vi "Filter-Init.vi"(5 "Filter":T1 {"IIR Filter Cluster"."Forward Coefficients" format="%.4f"; "IIR Filter Cluster"."Reverse Coefficients" format="%.4f"}, 9 "Sampling rate (Hz)":dbl, 11 "error in (no error)":errorcluster) -> (6 "Filter out":T1 {"IIR Filter Cluster"."Forward Coefficients" format="%.4f"; "IIR Filter Cluster"."Reverse Coefficients" format="%.4f"}, 15 "error out":errorcluster)   [LabVIEW 2020]
uses:
  Controls/Filter XCtl/Filter Data.ctl
  <vilib>/Analysis/3filter.llb/Filter Passband Type.ctl
  <vilib>/Analysis/NI_AALBase.lvlib
  Controls/Filter XCtl/Filter XCtl.xctl
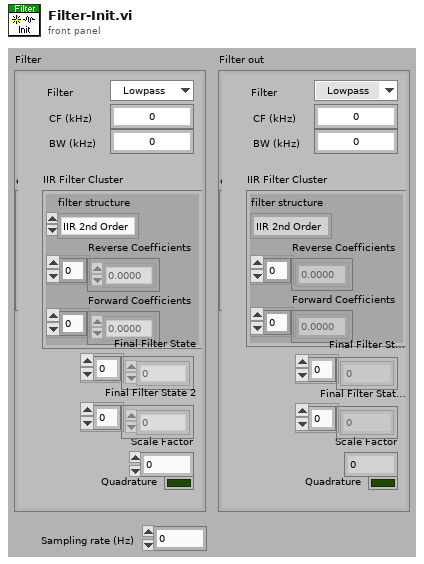
[diagram p1: front panel]
types:
  T1 = typedef "Filter XCtl.xctl/Filter Data.ctl" = cluster{"CF (kHz)":dbl, "BW (kHz)":dbl, "IIR Filter Cluster":cluster{"filter structure":enum32{"IIR 2nd Order", "IIR 4th Order"}, "Reverse Coefficients":dbl[], "Forward Coefficients":dbl[]}, "Final Filter State":dbl[], "Scale Factor":dbl, "Final Filter State 2":dbl[], "Quadrature":bool, "Type":enum16{"Lowpass", "Highpass", "Bandpass", "Bandstop", "OFF"}}
  T2 = enum16{"Lowpass", "Highpass", "Bandpass", "Bandstop", "OFF"}
  T3 = typedef "NI_AALBase.lvlib/Filter Passband Type.ctl" = enum32{"Lowpass", "Highpass", "Bandpass", "Bandstop"}
  T4 = cluster{"filter structure":enum32{"IIR 2nd Order", "IIR 4th Order"}, "Reverse Coefficients":dbl[], "Forward Coefficients":dbl[]}
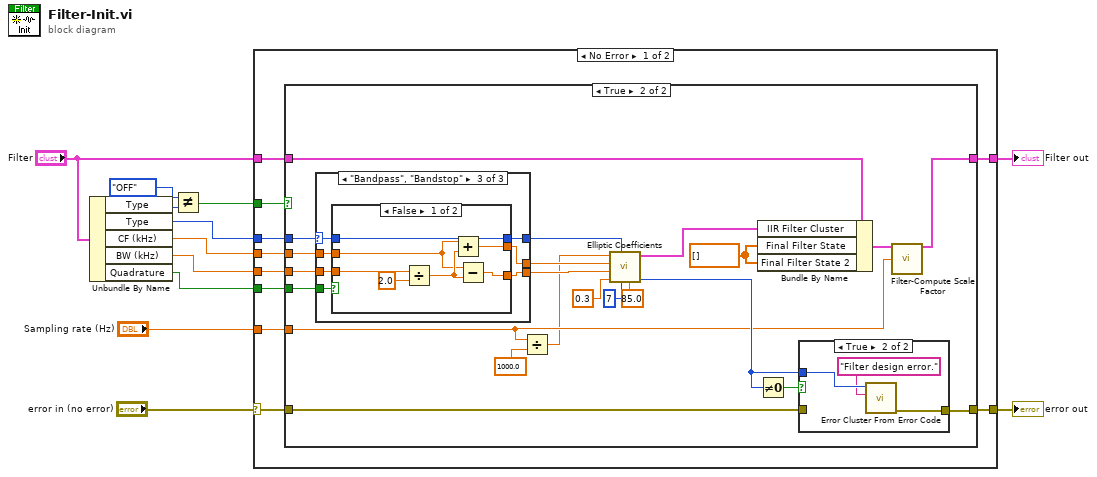
[diagram p0: block diagram]
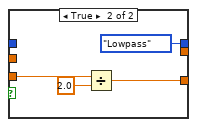
[diagram p6: hidden frame]
diagram:
  n1 = Unbundle By Name("Filter") -> ("Type"=w3:T2, "Type"=w11:T2, "CF (kHz)"=w8:dbl, "BW (kHz)"=w7:dbl, "Quadrature"=w4:bool)
  n2 = Not Equal?(x=T2."OFF", y=w3) -> (x != y?=w1:bool)
  n3 = case shown="No Error" "error in (no error)" {
    selector: "error in (no error)" -> [w15 w73]
    tunnel: w1 -> [w22 _]
    tunnel: w11 -> [w21 _]
    tunnel: "Sampling rate (Hz)" -> [w20 _]
    tunnel: "Filter" -> [w19 w74]
    tunnel: [w18 w74] -> w9
    tunnel: w8 -> [w17 _]
    tunnel: w7 -> [w16 _]
    tunnel: [w14 w73] -> w6
    tunnel: w4 -> [w13 _]
    frame No Error {
      n4 = case shown="True" w22 {
        tunnel: w21 -> [_ w31]
        tunnel: w20 -> [_ w33]
        tunnel: w19 -> [w24 w46]
        tunnel: [w24 w35] -> w18
        tunnel: w17 -> [_ w45]
        tunnel: w16 -> [_ w42]
        tunnel: w15 -> [w23 w40]
        tunnel: [w23 w39] -> w14
        tunnel: w13 -> [_ w28]
        frame False {
        }
        frame True {
          w30 = dbl[] [] ("Final Filter State")
          n5 = case shown="\"Bandpass\", \"Bandstop\"" w31 {
            selector: w31 -> [w51 w53 w56]
            tunnel: w45 -> [w52 w54 w58]
            tunnel: [w52 _ w59] -> w44
            tunnel: [_ w54 w60] -> w43
            tunnel: w42 -> [_ _ w61]
            tunnel: [w51 w53 w55] -> w29
            tunnel: w28 -> [_ _ w57]
            frame "Lowpass", Default {
            }
            frame "Highpass" {
            }
            frame "Bandpass", "Bandstop" {
              n6 = case shown="False" w57 {
                tunnel: w61 -> [w68 w71]
                tunnel: [w66 _] -> w60
                tunnel: [w65 w69] -> w59
                tunnel: w58 -> [w63 _]
                tunnel: w56 -> [w62 _]
                tunnel: [w62 Filter_Passband_Type."Lowpass" ("filter type")] -> w55
                frame False {
                  n7 = Divide(x=w68, y=2.0) -> (x/y=w64:dbl)
                  n8 = Add(x=w63, y=w64) -> (x+y=w66:dbl)
                  n9 = Subtract(x=w63, y=w64) -> (x-y=w65:dbl)
                }
                frame True {
                  n10 = Divide(x=w71, y=2.0) -> (x/y=w69:dbl)
                }
              }
            }
          }
          n11 = Divide(x=w33, y=1000.0) -> (x/y=w32:dbl)
          n12 = call <vilib>:"Elliptic Coefficients.vi"("stopband attenuation (dB)"=85.0, "order"=7, "filter type"=w29, "passband ripple (dB)"=0.3, "low cutoff freq: fl"=w44, "high cutoff freq: fh"=w43, "sampling freq: fs"=w32) -> ("error"=w38:i32, "IIR Filter Cluster"=w37:T4)  [unwired: 3 in]
          n13 = Bundle By Name(cluster=w46, "IIR Filter Cluster"=w37, "Final Filter State"=w30, "Final Filter State 2"=w30) -> (w36:T1)
          n14 = Not Equal To 0?(x=w38) -> (x != 0?=w41:bool)
          n15 = case shown="True" w41 {
            tunnel: [w47 w49] -> w39
            tunnel: w40 -> [w47 _]
            tunnel: w38 -> [_ w50]
            frame False {
            }
            frame True {
              n16 = call <vilib>:"Error Cluster From Error Code.vi"("error message (\"\")"="Filter design error." ("error message (\"\")"), "error code (0)"=w50) -> ("error out"=w49:errorcluster)  [unwired: 7 in]
            }
          }
          n17 = call "Filter-Compute Scale Factor.vi"("Filter"=w36, "Sampling Rate (Hz)"=w33) -> ("Filter out"=w35:T1)  [unwired: 12 in, 1 out]
        }
      }
    }
    frame Error {
    }
  }
  "error out" <- w6
  "Filter out" <- w9
